vi "Define_Best_Crossconnected_Pair-1.vi"(3 "[IN] Indicies of Cross\nconnected Points":i32[](array[numeric]), 5 "[IN] Tracks":dbl[][](array[numeric])) -> (1 "[OUT] Smallest Pair":i32)   [LabVIEW 2013]
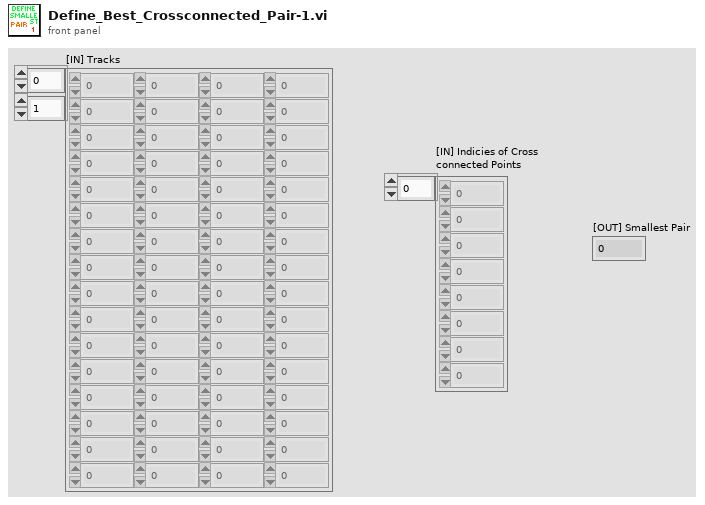
[diagram p1: front panel]
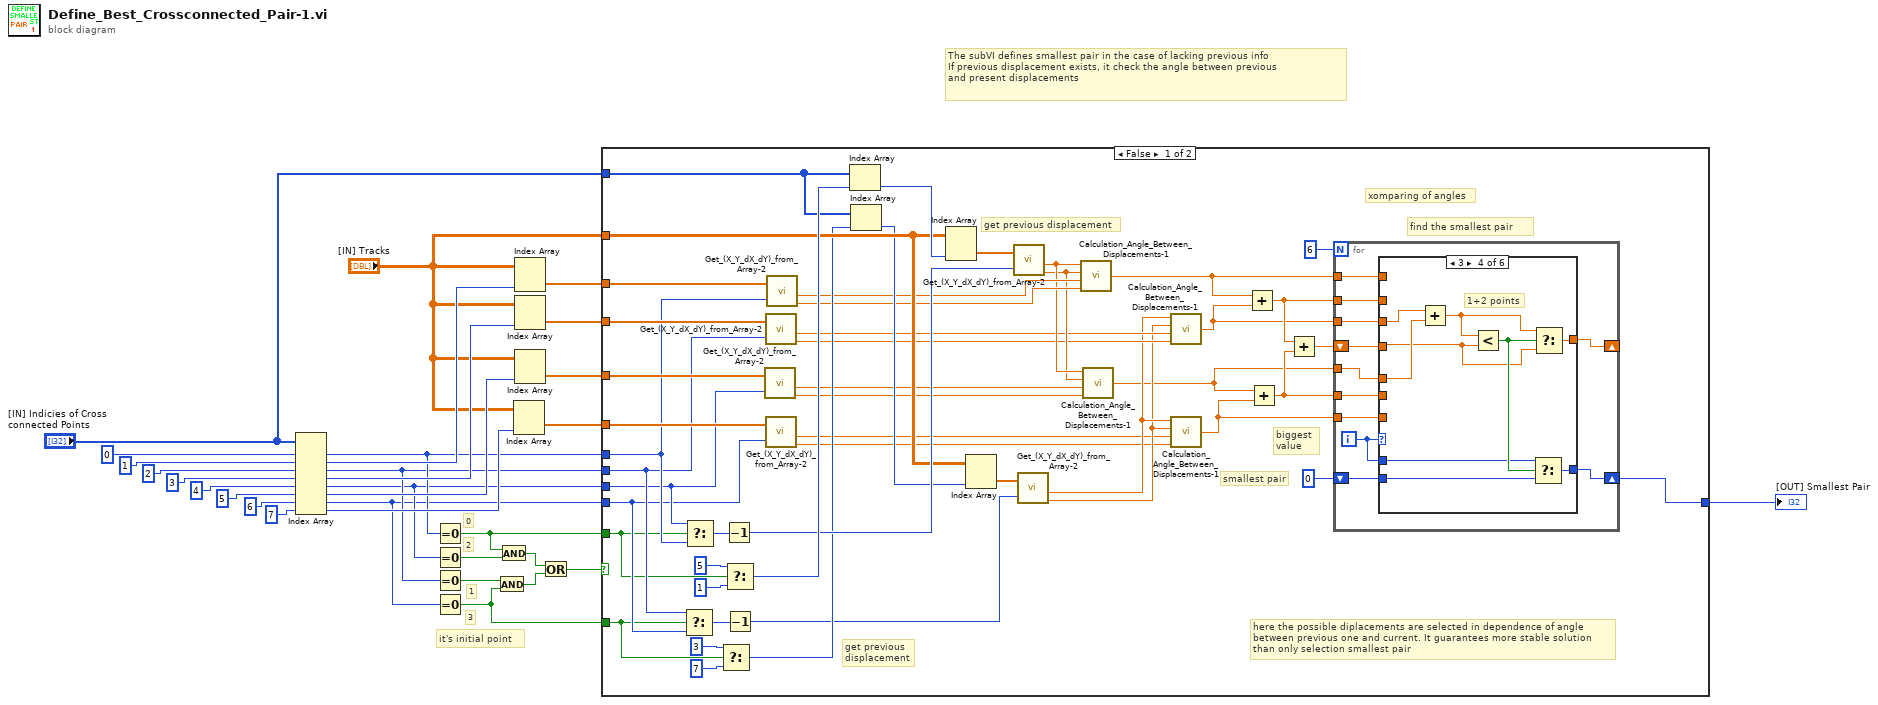
[diagram p0: block diagram]
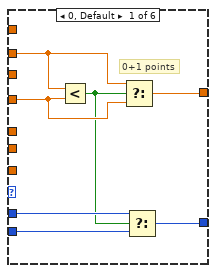
[diagram p2: hidden frame]
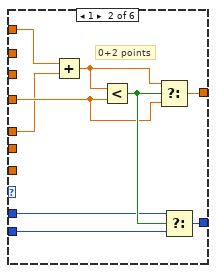
[diagram p3: hidden frame]
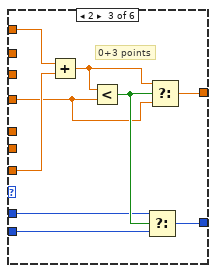
[diagram p4: hidden frame]
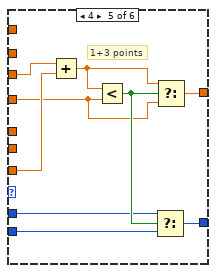
[diagram p5: hidden frame]
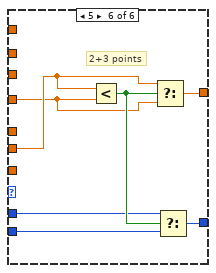
[diagram p6: hidden frame]
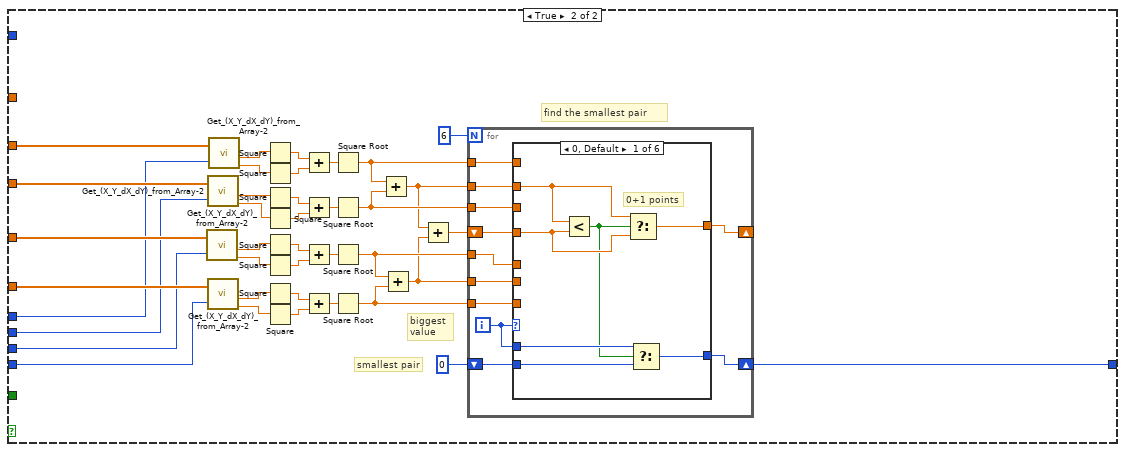
[diagram p7: hidden frame]
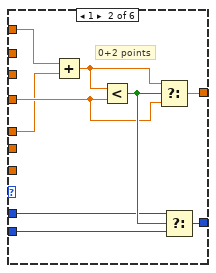
[diagram p8: hidden frame]
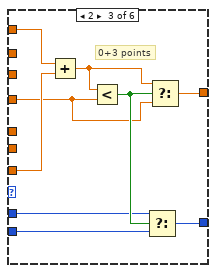
[diagram p9: hidden frame]
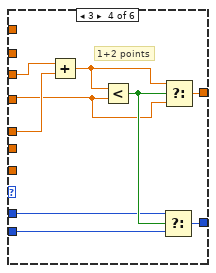
[diagram p10: hidden frame]
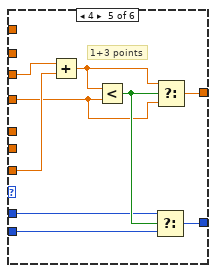
[diagram p11: hidden frame]
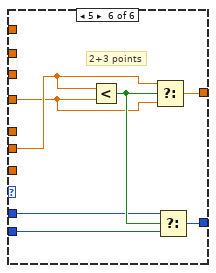
[diagram p12: hidden frame]
diagram:
  # "3"
  # "1"
  # "2"
  # "0"
  # "it's initial point"
  # "The subVI defines smallest pair in the case of lacking previous info\nIf previous displacement exists, it check the angle between previous \nand present displacements"
  n1 = Index Array(array="[IN] Indicies of Cross\nconnected Points", index #1=0 ("index"), index #2=1 ("index"), index #3=2 ("index"), index #4=3 ("index"), index #5=4 ("index"), index #6=5 ("index"), index #7=6 ("index"), index #8=7 ("index")) -> (element #1=w13:i32, element #2=w15:i32, element #3=w12:i32, element #4=w22:i32, element #5=w11:i32, element #6=w21:i32, element #7=w10:i32, element #8=w20:i32)
  n2 = Equal To 0?(x=w13) -> (x = 0?=w6:bool)
  n3 = Equal To 0?(x=w11) -> (x = 0?=w7:bool)
  n4 = Equal To 0?(x=w12) -> (x = 0?=w5:bool)
  n5 = Equal To 0?(x=w10) -> (x = 0?=w4:bool)
  n6 = And(x=w5, y=w4) -> (x .and. y?=w8:bool)
  n7 = And(x=w6, y=w7) -> (x .and. y?=w9:bool)
  n8 = Index Array(array="[IN] Tracks", index (col)=w20) -> (element=w16:dbl[])  [unwired: 1 in]
  n9 = Index Array(array="[IN] Tracks", index (col)=w15) -> (element=w19:dbl[])  [unwired: 1 in]
  n10 = Index Array(array="[IN] Tracks", index (col)=w22) -> (element=w18:dbl[])  [unwired: 1 in]
  n11 = Index Array(array="[IN] Tracks", index (col)=w21) -> (element=w17:dbl[])  [unwired: 1 in]
  n12 = Or(x=w9, y=w8) -> (x .or. y?=w3:bool)
  n13 = case shown="False" w3 {
    tunnel: w19 -> [w76 w177]
    tunnel: w18 -> [w75 w176]
    tunnel: w17 -> [w74 w175]
    tunnel: w16 -> [w73 w174]
    tunnel: [w32 w165] -> w14
    tunnel: w13 -> [w72 w164]
    tunnel: w12 -> [w71 w163]
    tunnel: w11 -> [w70 w162]
    tunnel: w10 -> [w69 w161]
    tunnel: w6 -> [w68 _]
    tunnel: w4 -> [w63 _]
    tunnel: "[IN] Tracks" -> [w57 _]
    tunnel: "[IN] Indicies of Cross\nconnected Points" -> [w58 _]
    frame False {
      # "here the possible diplacements are selected in dependence of angle\nbetween previous one and current. It guarantees more stable solution\nthan only selection smallest pair"
      # "xomparing of angles"
      # "smallest pair"
      # "biggest \nvalue"
      # "find the smallest pair"
      # "get previous displacement"
      # "get previous \ndisplacement"
      n14 = Select(t=w71, s=w63, f=w69) -> (s? t:f=w77:i32)
      n15 = Select(t=w70, s=w68, f=w72) -> (s? t:f=w78:i32)
      n16 = Select(t=3 ("index"), s=w63, f=7 ("index")) -> (s? t:f=w54:i32)
      n17 = Decrement(x=w78) -> (x-1=w59:i32)
      n18 = Select(t=5 ("index"), s=w68, f=1 ("index")) -> (s? t:f=w62:i32)
      n19 = Decrement(x=w77) -> (x-1=w31:i32)
      n20 = call "Get_(X_Y_dX_dY)_from_Array-2.vi"("(X,Y,dX,dY)"=w74, "Index of Displacement"=w70) -> ("dX"=w49:dbl, "dY"=w48:dbl)  [unwired: 2 out]
      n21 = call "Get_(X_Y_dX_dY)_from_Array-2.vi"("(X,Y,dX,dY)"=w75, "Index of Displacement"=w71) -> ("dX"=w47:dbl, "dY"=w46:dbl)  [unwired: 2 out]
      n22 = call "Get_(X_Y_dX_dY)_from_Array-2.vi"("(X,Y,dX,dY)"=w73, "Index of Displacement"=w69) -> ("dX"=w43:dbl, "dY"=w42:dbl)  [unwired: 2 out]
      n23 = call "Get_(X_Y_dX_dY)_from_Array-2.vi"("(X,Y,dX,dY)"=w76, "Index of Displacement"=w72) -> ("dX"=w53:dbl, "dY"=w52:dbl)  [unwired: 2 out]
      n24 = Index Array(array=w58, index=w62) -> (element=w61:i32)
      n25 = Index Array(array=w58, index=w54) -> (element=w56:i32)
      n26 = Index Array(array=w57, index (col)=w61) -> (element=w60:dbl[])  [unwired: 1 in]
      n27 = Index Array(array=w57, index (col)=w56) -> (element=w55:dbl[])  [unwired: 1 in]
      n28 = call "Get_(X_Y_dX_dY)_from_Array-2.vi"("(X,Y,dX,dY)"=w60, "Index of Displacement"=w59) -> ("dX"=w51:dbl, "dY"=w50:dbl)  [unwired: 2 out]
      n29 = call "Get_(X_Y_dX_dY)_from_Array-2.vi"("(X,Y,dX,dY)"=w55, "Index of Displacement"=w31) -> ("dX"=w45:dbl, "dY"=w44:dbl)  [unwired: 2 out]
      n30 = call "Calculation_Angle_Between_Displacements-1.vi"("dY 2"=w52, "dX 2"=w53, "dY 1"=w50, "dX 1"=w51) -> ("angle in degrees"=w36:dbl)
      n31 = call "Calculation_Angle_Between_Displacements-1.vi"("dY 2"=w48, "dX 2"=w49, "dY 1"=w50, "dX 1"=w51) -> ("angle in degrees"=w33:dbl)
      n32 = call "Calculation_Angle_Between_Displacements-1.vi"("dY 2"=w46, "dX 2"=w47, "dY 1"=w44, "dX 1"=w45) -> ("angle in degrees"=w35:dbl)
      n33 = call "Calculation_Angle_Between_Displacements-1.vi"("dY 2"=w42, "dX 2"=w43, "dY 1"=w44, "dX 1"=w45) -> ("angle in degrees"=w34:dbl)
      n34 = Add(x=w36, y=w35) -> (x+y=w38:dbl)
      n35 = Add(x=w33, y=w34) -> (x+y=w37:dbl)
      n36 = Add(x=w38, y=w37) -> (x+y=w40:dbl)
      n37 = for {
        N: 6 -> [_]
        tunnel: w36 -> [w87]
        tunnel: w35 -> [w86]
        tunnel: w33 -> [w81]
        tunnel: w34 -> [w80]
        shift-right: [w84] -> _
        shift-left: w40 -> [w89]
        tunnel: w38 -> [w88]
        tunnel: w37 -> [w79]
        shift-right: [w82] -> w32
        shift-left: 0 -> [w83]
        i -> [w85]
        n38 = case shown="3" w85 {
          tunnel: w89 -> [w95 w100 w108 w117 w126 w135]
          tunnel: w88 -> [w96 _ _ _ _ _]
          tunnel: w87 -> [_ w105 w110 _ _ _]
          tunnel: w86 -> [_ _ _ w119 w128 _]
          tunnel: w85 -> [w93 w102 w112 w121 w125 w138]
          tunnel: [w94 w97 w107 w116 w130 w134] -> w84
          tunnel: w83 -> [w92 w101 w111 w120 w124 w137]
          tunnel: [w91 w103 w106 w115 w129 w133] -> w82
          tunnel: w81 -> [_ w98 _ w118 _ _]
          tunnel: w80 -> [_ _ w109 _ w127 _]
          tunnel: w79 -> [_ _ _ _ _ w136]
          frame 0, Default {
            # "0+1 points"
            n39 = Less?(x=w96, y=w95) -> (x < y?=w90:bool)
            n40 = Select(t=w96, s=w90, f=w95) -> (s? t:f=w94:dbl)
            n41 = Select(t=w93, s=w90, f=w92) -> (s? t:f=w91:i32)
          }
          frame 1 {
            # "0+2 points"
            n42 = Add(x=w105, y=w98) -> (x+y=w99:dbl)
            n43 = Less?(x=w99, y=w100) -> (x < y?=w104:bool)
            n44 = Select(t=w99, s=w104, f=w100) -> (s? t:f=w97:dbl)
            n45 = Select(t=w102, s=w104, f=w101) -> (s? t:f=w103:i32)
          }
          frame 2 {
            # "0+3 points"
            n46 = Add(x=w110, y=w109) -> (x+y=w113:dbl)
            n47 = Less?(x=w113, y=w108) -> (x < y?=w114:bool)
            n48 = Select(t=w112, s=w114, f=w111) -> (s? t:f=w106:i32)
            n49 = Select(t=w113, s=w114, f=w108) -> (s? t:f=w107:dbl)
          }
          frame 3 {
            # "1+2 points"
            n50 = Add(x=w119, y=w118) -> (x+y=w122:dbl)
            n51 = Less?(x=w122, y=w117) -> (x < y?=w123:bool)
            n52 = Select(t=w121, s=w123, f=w120) -> (s? t:f=w115:i32)
            n53 = Select(t=w122, s=w123, f=w117) -> (s? t:f=w116:dbl)
          }
          frame 4 {
            # "1+3 points"
            n54 = Add(x=w128, y=w127) -> (x+y=w131:dbl)
            n55 = Less?(x=w131, y=w126) -> (x < y?=w132:bool)
            n56 = Select(t=w125, s=w132, f=w124) -> (s? t:f=w129:i32)
            n57 = Select(t=w131, s=w132, f=w126) -> (s? t:f=w130:dbl)
          }
          frame 5 {
            # "2+3 points"
            n58 = Less?(x=w136, y=w135) -> (x < y?=w139:bool)
            n59 = Select(t=w136, s=w139, f=w135) -> (s? t:f=w134:dbl)
            n60 = Select(t=w138, s=w139, f=w137) -> (s? t:f=w133:i32)
          }
        }
      }
    }
    frame True {
      # "smallest pair"
      # "biggest \nvalue"
      # "find the smallest pair"
      n61 = call "Get_(X_Y_dX_dY)_from_Array-2.vi"("(X,Y,dX,dY)"=w175, "Index of Displacement"=w162) -> ("dX"=w169:dbl, "dY"=w168:dbl)  [unwired: 2 out]
      n62 = call "Get_(X_Y_dX_dY)_from_Array-2.vi"("(X,Y,dX,dY)"=w176, "Index of Displacement"=w163) -> ("dX"=w171:dbl, "dY"=w170:dbl)  [unwired: 2 out]
      n63 = call "Get_(X_Y_dX_dY)_from_Array-2.vi"("(X,Y,dX,dY)"=w174, "Index of Displacement"=w161) -> ("dX"=w167:dbl, "dY"=w166:dbl)  [unwired: 2 out]
      n64 = call "Get_(X_Y_dX_dY)_from_Array-2.vi"("(X,Y,dX,dY)"=w177, "Index of Displacement"=w164) -> ("dX"=w173:dbl, "dY"=w172:dbl)  [unwired: 2 out]
      n65 = Square(x=w173) -> (x^2=w160:dbl)
      n66 = Square(x=w172) -> (x^2=w159:dbl)
      n67 = Square(x=w171) -> (x^2=w157:dbl)
      n68 = Square(x=w170) -> (x^2=w156:dbl)
      n69 = Square(x=w169) -> (x^2=w154:dbl)
      n70 = Square(x=w168) -> (x^2=w153:dbl)
      n71 = Square(x=w167) -> (x^2=w151:dbl)
      n72 = Square(x=w166) -> (x^2=w150:dbl)
      n73 = Add(x=w160, y=w159) -> (x+y=w158:dbl)
      n74 = Add(x=w157, y=w156) -> (x+y=w155:dbl)
      n75 = Add(x=w154, y=w153) -> (x+y=w152:dbl)
      n76 = Add(x=w151, y=w150) -> (x+y=w149:dbl)
      n77 = Square Root(x=w158) -> (sqrt(x)=w147:dbl)
      n78 = Square Root(x=w155) -> (sqrt(x)=w146:dbl)
      n79 = Square Root(x=w152) -> (sqrt(x)=w145:dbl)
      n80 = Square Root(x=w149) -> (sqrt(x)=w144:dbl)
      n81 = Add(x=w147, y=w146) -> (x+y=w141:dbl)
      n82 = Add(x=w145, y=w144) -> (x+y=w140:dbl)
      n83 = Add(x=w141, y=w140) -> (x+y=w143:dbl)
      n84 = for {
        N: 6 -> [_]
        tunnel: w147 -> [w186]
        tunnel: w146 -> [w185]
        tunnel: w145 -> [w180]
        tunnel: w144 -> [w179]
        shift-right: [w183] -> _
        shift-left: w143 -> [w188]
        tunnel: w141 -> [w187]
        tunnel: w140 -> [w178]
        shift-right: [w181] -> w165
        shift-left: 0 -> [w182]
        i -> [w184]
        n85 = case shown="0, Default" w184 {
          tunnel: w188 -> [w194 w199 w207 w216 w225 w234]
          tunnel: w187 -> [w195 _ _ _ _ _]
          tunnel: w186 -> [_ w204 w209 _ _ _]
          tunnel: w185 -> [_ _ _ w218 w227 _]
          tunnel: w184 -> [w192 w201 w211 w220 w224 w237]
          tunnel: [w193 w196 w206 w215 w229 w233] -> w183
          tunnel: w182 -> [w191 w200 w210 w219 w223 w236]
          tunnel: [w190 w202 w205 w214 w228 w232] -> w181
          tunnel: w180 -> [_ w197 _ w217 _ _]
          tunnel: w179 -> [_ _ w208 _ w226 _]
          tunnel: w178 -> [_ _ _ _ _ w235]
          frame 0, Default {
            # "0+1 points"
            n86 = Less?(x=w195, y=w194) -> (x < y?=w189:bool)
            n87 = Select(t=w195, s=w189, f=w194) -> (s? t:f=w193:dbl)
            n88 = Select(t=w192, s=w189, f=w191) -> (s? t:f=w190:i32)
          }
          frame 1 {
            # "0+2 points"
            n89 = Add(x=w204, y=w197) -> (x+y=w198:dbl)
            n90 = Less?(x=w198, y=w199) -> (x < y?=w203:bool)
            n91 = Select(t=w198, s=w203, f=w199) -> (s? t:f=w196:dbl)
            n92 = Select(t=w201, s=w203, f=w200) -> (s? t:f=w202:i32)
          }
          frame 2 {
            # "0+3 points"
            n93 = Add(x=w209, y=w208) -> (x+y=w212:dbl)
            n94 = Less?(x=w212, y=w207) -> (x < y?=w213:bool)
            n95 = Select(t=w211, s=w213, f=w210) -> (s? t:f=w205:i32)
            n96 = Select(t=w212, s=w213, f=w207) -> (s? t:f=w206:dbl)
          }
          frame 3 {
            # "1+2 points"
            n97 = Add(x=w218, y=w217) -> (x+y=w221:dbl)
            n98 = Less?(x=w221, y=w216) -> (x < y?=w222:bool)
            n99 = Select(t=w220, s=w222, f=w219) -> (s? t:f=w214:i32)
            n100 = Select(t=w221, s=w222, f=w216) -> (s? t:f=w215:dbl)
          }
          frame 4 {
            # "1+3 points"
            n101 = Add(x=w227, y=w226) -> (x+y=w230:dbl)
            n102 = Less?(x=w230, y=w225) -> (x < y?=w231:bool)
            n103 = Select(t=w224, s=w231, f=w223) -> (s? t:f=w228:i32)
            n104 = Select(t=w230, s=w231, f=w225) -> (s? t:f=w229:dbl)
          }
          frame 5 {
            # "2+3 points"
            n105 = Less?(x=w235, y=w234) -> (x < y?=w238:bool)
            n106 = Select(t=w235, s=w238, f=w234) -> (s? t:f=w233:dbl)
            n107 = Select(t=w237, s=w238, f=w236) -> (s? t:f=w232:i32)
          }
        }
      }
    }
  }
  "[OUT] Smallest Pair" <- w14
